vi "Is File an LLB.vi"(8 "error in (no error)":errorcluster, 11 "path":path) -> (0 "error out":errorcluster, 3 "Is LLB?":bool)   [LabVIEW 2020, in "NI_FileType.lvlib"]
doc: "Returns TRUE if this file is an LLB."
uses:
  NI_FileType.lvlib
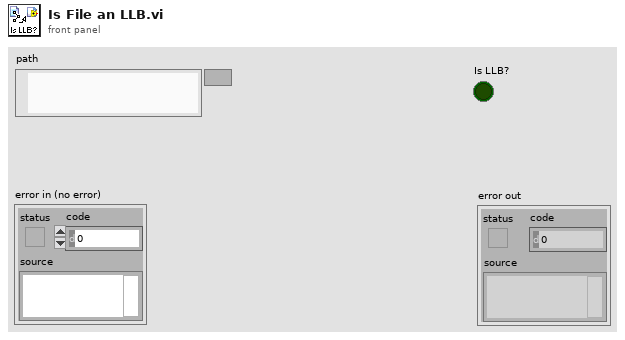
[diagram p1: front panel]
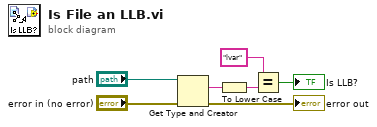
[diagram p0: block diagram]
diagram:
  n1 = Get Type and Creator(4:"error in (no error)", 7:"path") -> (0:→"error out":errorcluster, 2:w4:string)  [unwired: 2 out]
  n2 = To Lower Case(string=w4) -> (all lower case string=w3:string)
  n3 = Equal?(x="lvar", y=w3) -> (x = y?=→"Is LLB?":bool)
